vi "ScottSight2.0_Button_Cycle.vi"() -> ()   [LabVIEW 2013]
panel:
  out "Count Cyle":dbl
  out "Numeric":dbl
  out "Waveform Chart":dynamicdata(graph)
  in  "Samples":dbl
  in  "Rate":dbl
  in  "Stop":bool
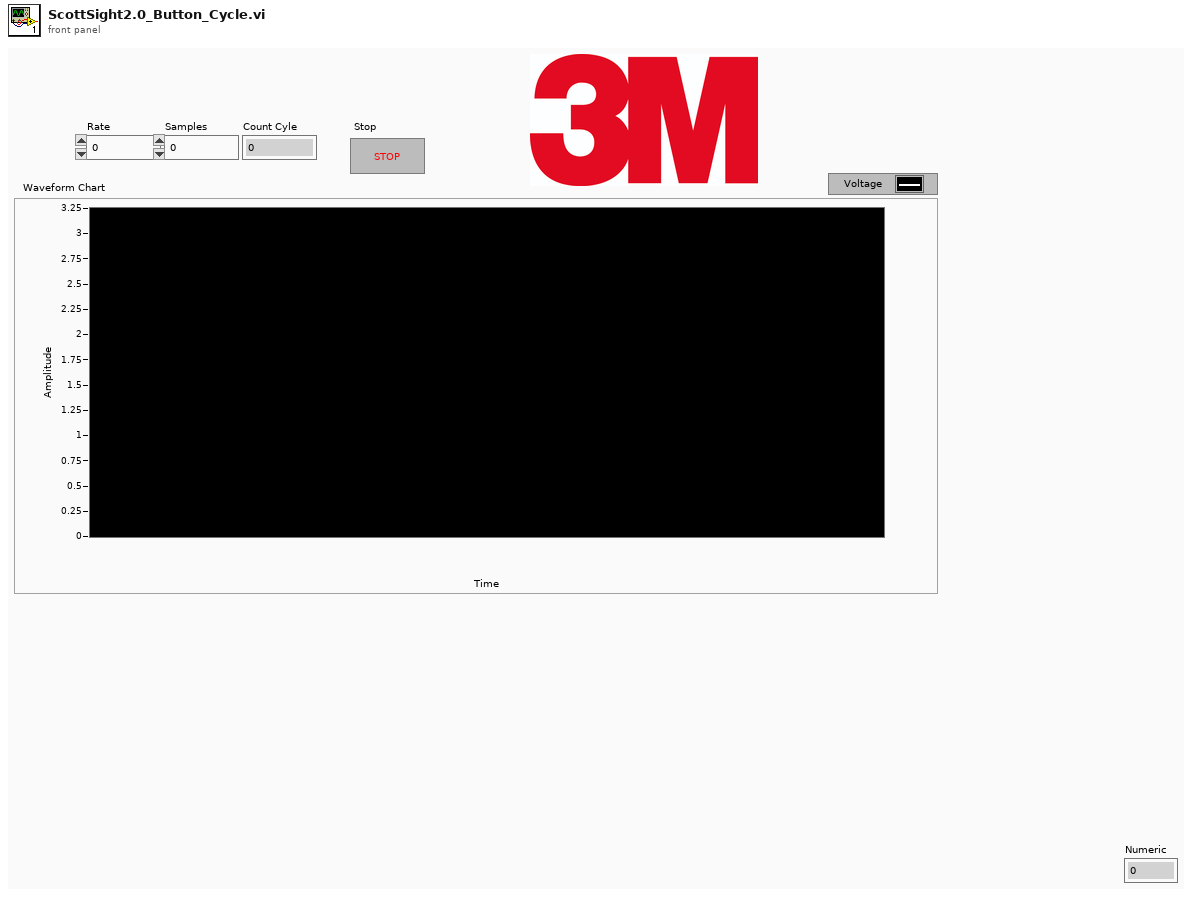
[diagram p1: front panel]
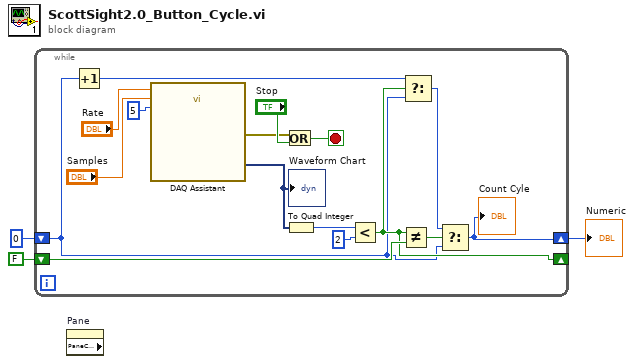
[diagram p0: block diagram]
diagram:
  n1 = while {
    shift-right: [w4] -> w1
    shift-left: 0 -> [w5]
    shift-right: [w6] -> _
    shift-left: FALSE -> [w7]
    stop <- w18 stop-if-true
    n2 = Increment(x=w5) -> (x+1=w10:i32)
    n3 = call "DAQ Assistant"("rate"="Rate", "number of samples"="Samples", "timeout (s)"=5) -> ("data"=w12:dynamicdata, "error out"=w14:errorcluster)  [unwired: 13 in, 2 out]
    "Waveform Chart" <- w12
    n4 = Or(x=w14, y="Stop") -> (x .or. y?=w18:bool)
    n5 = To Quad Integer(1:w12) -> (0:w11:i64)
    n6 = Less?(x=w11, y=2) -> (x < y?=w6:bool)
    n7 = Not Equal?(x=w6, y=w7) -> (x != y?=w8:bool)
    n8 = Select(t=w10, s=w6, f=w5) -> (s? t:f=w9:i32)
    n9 = Select(t=w9, s=w8, f=w5) -> (s? t:f=w4:i32)
    "Count Cyle" <- w4
  }
  "Numeric" <- w1
  n10 = property on="Pane" class="Pane" props=["PaneColor"]() -> ()  [unwired: 2 in, 3 out]
